vi "Disabled - Load From Constant File (SubVI).vi"(9 "File Name":string, 10 "Robot Path":string, 11 "Trigger Reload":bool) -> (2 "error out":errorcluster, 3 "Array":string[](array[string]))   [LabVIEW 2019]
doc: "Loads constants from a file into an array."
panel:
  # "Inputs"
  # "Outputs"
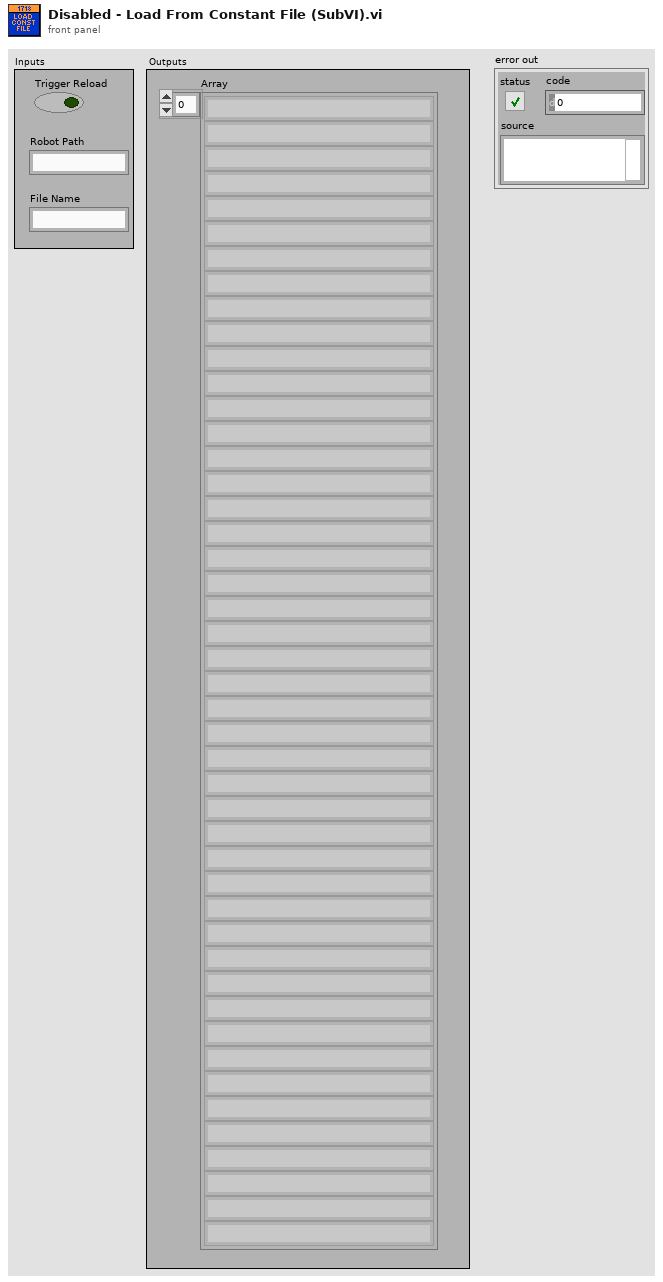
[diagram p1: front panel]
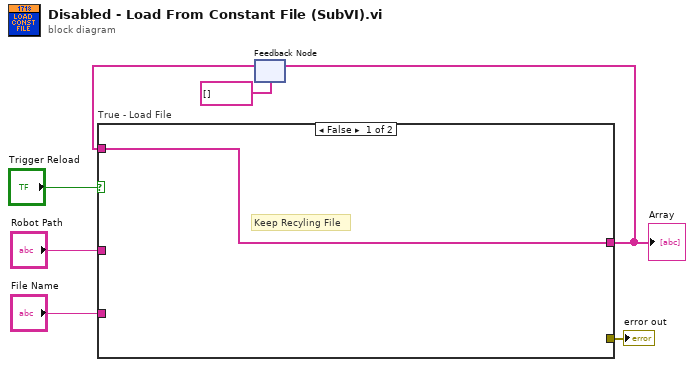
[diagram p0: block diagram]
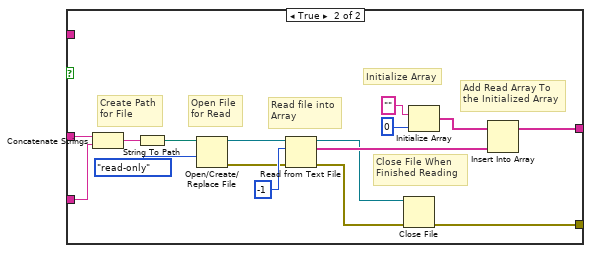
[diagram p2: hidden frame]
diagram:
  n1 = feedback #1(string[] []) -> (w2:string[])
  n2 = case "True - Load File" shown="False" "Trigger Reload" {
    tunnel: [w8 w23] -> w7
    tunnel: w2 -> [w8 _]
    tunnel: "Robot Path" -> [_ w13]
    tunnel: "File Name" -> [_ w12]
    tunnel: [_ w9] -> w1
    frame False {
      # "Keep Recyling File"
    }
    frame True {
      # "Create Path\nfor File"
      # "Open File\nfor Read"
      # "Read file into\nArray"
      # "Close File When\nFinished Reading"
      # "Add Read Array To\nthe Initialized Array"
      # "Initialize Array"
      n3 = Concatenate Strings(w13, w12) -> (w18:string)
      n4 = String To Path(string=w18) -> (path=w17:path)
      n5 = Open/Create/Replace File(file path (use dialog)=w17, access (0:read/write)=enum16{"read/write", "read-only", "write-only"}."read-only") -> (refnum out=w22:refnum<file>, error out=w21:errorcluster)  [unwired: 1 in, 4 out]
      n6 = Read from Text File(file (use dialog)=w22, count=-1, error in=w21) -> (refnum out=w11:refnum<file>, text=w19:string[], error out=w10:errorcluster)  [unwired: 2 out]
      n7 = Close File(refnum=w11, error in=w10) -> (error out=w9:errorcluster)  [unwired: 1 out]
      n8 = Initialize Array("" ("string"), 0 ("dimension size")) -> (w20:string[])
      n9 = Insert Into Array(array=w20, new element=w19) -> (w23:string[])  [unwired: 1 in]
    }
  }
  "Array" <- w7
  "error out" <- w1
  n10 = feedback-in #1(w7) -> ()
